vi "Open TCP Session.vi"(7 "Slave ID (255)":u8=255, 8 "error in (no error)":errorcluster, 9 "Timeout (10000)":i32=10000, 10 "Port (502)":u16=502, 11 "IP Address":string="localhost") -> (0 "error out":errorcluster, 3 "MB_TCP session":refnum<class "MB_Master_TCP.lvclass">)   [LabVIEW 2023, in "Jiaxin_Stepper_Controller.lvlib" / "MB Master.lvlib" / "MB_Master_TCP.lvclass"]
doc: "Opens a new modbus session and establish the TCP connection. Note that the slave ID is set to the default of 0xFF. Slave ID can be changed later via the property node \"Slave ID\"."
uses:
  MB_Master_TCP.lvclass
  MB_ADU/MB_ADU.lvclass/MB_ADU.ctl
  MB_ADU_TCP/MB_ADU_TCP.lvclass/MB_ADU_TCP.ctl
  MB_Master_TCP.lvclass/MB_Master_TCP.ctl
  MB_ADU/Build ADU.vi
  MB_ADU_TCP/MB_ADU_TCP.lvclass
  C:/Users/quantum/Documents/SinglePhotonUI/Plasmionique/MB Master/MB_ADU/MB_ADU.lvclass
  Core.vi
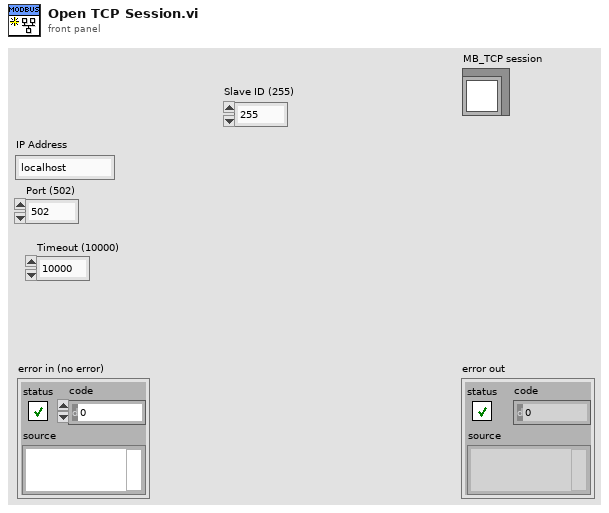
[diagram p1: front panel]
types:
  T1 = cluster{"IP Address":string, "Port":u16, "Timeout":i32, "Notifier":refnum<notifier>}
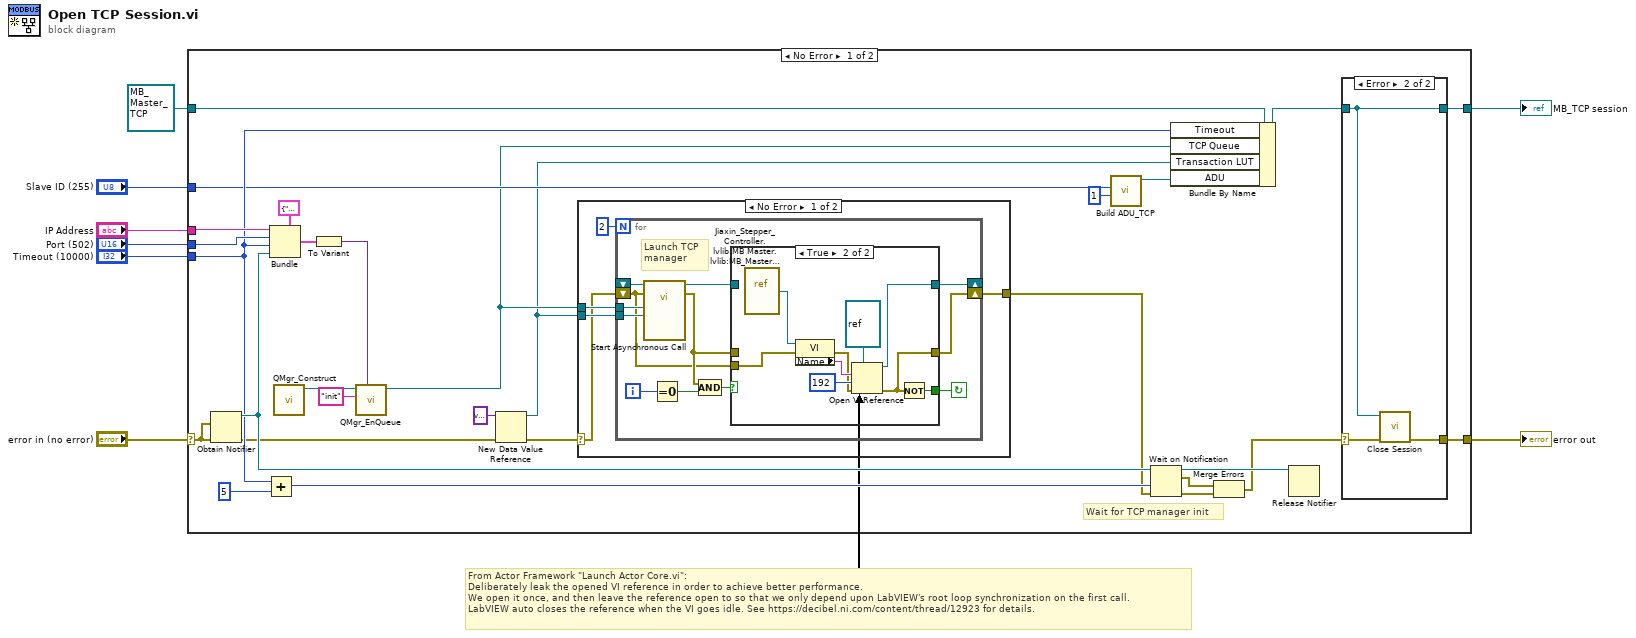
[diagram p0: block diagram]
diagram:
  # "From Actor Framework \"Launch Actor Core.vi\":\nDeliberately leak the opened VI reference in order to achieve better performance.\nWe open it once, and then leave the reference open to so that we only depend upon LabVIEW's root loop synchronization on the first call.\nLabVIEW auto closes the reference when the VI goes idle. See https://decibel.ni.com/content/thread/12923 for details."
  n1 = case shown="No Error" "error in (no error)" {
    selector: "error in (no error)" -> [w23 w73]
    tunnel: [w24 w73] -> w7
    tunnel: [w26 w72] -> w5
    tunnel: refnum<class "MB_Master_TCP.lvclass"> refnum ("MB_Master_TCP in") -> [w37 w72]
    tunnel: "IP Address" -> [w33 _]
    tunnel: "Port (502)" -> [w32 _]
    tunnel: "Timeout (10000)" -> [w21 _]
    tunnel: "Slave ID (255)" -> [w13 _]
    frame No Error {
      # "Wait for TCP manager init"
      n2 = Obtain Notifier(notification data type=w23, error in (no error)=w23) -> (notifier out=w29:refnum<notifier>, error out=w14:errorcluster)  [unwired: 2 in, 1 out]
      n3 = Add(x=w21, y=5) -> (x+y=w19:i32)
      n4 = Bundle(cluster=T1 {"IP Address"="", "Port"=502, "Timeout"=10000, "Notifier"=refnum}, "IP Address"=w33, "Port"=w32, "Timeout"=w21, "Notifier"=w29) -> (w30:T1)
      n5 = call "QMgr_Construct.vi"() -> ("queue out"=w17:refnum<queue>)  [unwired: 11 in]
      n6 = To Variant(anything=w30) -> (Variant=w15:variant)
      n7 = call "QMgr_EnQueue.vi"("Data"=w15, "Command"="init" ("cmd"), "queue in"=w17) -> ("queue out"=w12:refnum<queue>)  [unwired: 8 in]
      n8 = New Data Value Reference(data value=variant ("variant"), error in=w14) -> (data value reference=w11:refnum<data-value>, error out=w9:errorcluster)
      n9 = case shown="No Error" w9 {
        selector: w9 -> [w38 w66]
        tunnel: w12 -> [w41 _]
        tunnel: w11 -> [w40 _]
        tunnel: [w39 w66] -> w10
        frame No Error {
          n10 = for {
            N: 2 -> [_]
            shift-right: [w53] -> _
            shift-left: _ -> [w52]
            shift-right: [w47] -> w39
            shift-left: w38 -> [w43]
            tunnel: w41 -> [w45]
            tunnel: w40 -> [w44]
            i -> [w51]
            stop <- w48 continue-if-true
            # "Launch TCP\nmanager"
            n11 = call-by-ref "Start Asynchronous Call"(reference=w52, error in=w43, "Transaction LUT"=w44, "CMD Queue"=w45) -> (reference out=w54:refnum<vi>, error out=w46:errorcluster)  [unwired: 10 in]
            n12 = Equal To 0?(x=w51) -> (x = 0?=w50:bool)
            n13 = Compound Arithmetic op=AND(w46, w50) -> (w49:bool)
            n14 = case shown="True" w49 {
              tunnel: w54 -> [w56 _]
              tunnel: [w56 w61] -> w53
              tunnel: [_ w60] -> w48
              tunnel: [w55 w59] -> w47
              tunnel: w46 -> [w55 _]
              tunnel: w43 -> [_ w58]
              frame False {
              }
              frame True {
                n15 = vi-ref "Jiaxin_Stepper_Controller.lvlib:MB Master.lvlib:MB_Master_TCP.lvclass:Core.vi"() -> (w65:refnum<vi>)
                n16 = property class="VI"(reference=w65, error in=w58) -> (error out=w57:errorcluster, "Name"=w62:string)  [unwired: 1 out]
                n17 = Open VI Reference(type specifier VI Refnum (for type only)=refnum<vi> refnum, vi path=w62, options=192, error in (no error)=w57) -> (vi reference=w61:refnum<vi>, error out=w59:errorcluster)  [unwired: 2 in]
                n18 = Not(x=w59) -> (.not. x?=w60:bool)
              }
            }
          }
        }
        frame Error {
        }
      }
      n19 = call "Build ADU_TCP.vi"("Transaction ID"=u16 1, "Slave ID"=w13) -> ("MB_ADU_TCP out"=w36:refnum<class "MB_ADU_TCP.lvclass">)  [unwired: 8 in, 1 out]
      n20 = Wait on Notification(notifier=w29, timeout in ms (-1)=w19, error in (no error)=w10) -> (notifier out=w22:refnum<notifier>, notification=w27:errorcluster, error out=w28:errorcluster)  [unwired: 1 in, 1 out]
      n21 = Bundle By Name(cluster=w37, "Timeout"=w21, "TCP Queue"=w12, "Transaction LUT"=w11, "ADU"=w36) -> (w25:refnum<class "MB_Master_TCP.lvclass">)
      n22 = Merge Errors(w27, w28) -> (w18:errorcluster)
      n23 = Release Notifier(notifier=w22) -> ()  [unwired: 2 in, 3 out]
      n24 = case shown="Error" w18 {
        selector: w18 -> [w67 w69]
        tunnel: [w68 w70] -> w26
        tunnel: w25 -> [w68 w70]
        tunnel: [w67 w71] -> w24
        frame No Error {
        }
        frame Error {
          n25 = call-dynamic "Close Session.vi"("error in (no error)"=w69, "MB TCP session"=w70) -> ("error out"=w71:errorcluster)  [unwired: 9 in]
        }
      }
    }
    frame Error {
    }
  }
  "error out" <- w7
  "MB_TCP session" <- w5
